vi "use python.vi"() -> ()   [LabVIEW 2024]
panel:
  in  "b":i32
  in  "a":i32
  out "a + b":i32
  in  "函数名称":string
  in  "模块路径":path
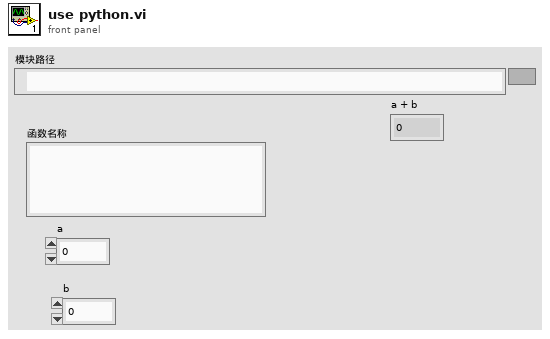
[diagram p1: front panel]
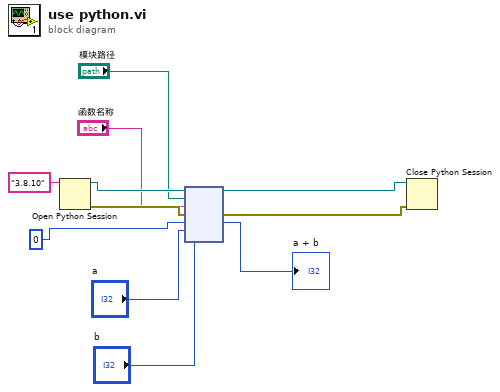
[diagram p0: block diagram]
diagram:
  n1 = Open Python Session(python version="3.8.10" ("Python版本")) -> (session out=w11:refnum<k35>, error out=w8:errorcluster)  [unwired: 2 in]
  n2 = node(w11, "模块路径", "函数名称", w8, 0 ("a + b"), "a", "b") -> (w10:refnum<k35>, w9:errorcluster, →"a + b":i32)  [unwired: 2 in, 2 out]
  n3 = Close Python Session(session in=w10, error in=w9) -> ()  [unwired: 1 out]
